vi "Configure Return Delay.vi"(8 "error in (no error)":errorcluster, 9 "Return Delay (500 microseconds)":sgl=500.0, 10 "Motor ID (0)":u8, 11 "Dynamixel Motor VISA in":refnum<class "Dynamixel Motor VISA.lvclass">) -> (0 "error out":errorcluster, 3 "Dynamixel Motor VISA out":refnum<class "Dynamixel Motor VISA.lvclass">)   [LabVIEW 2016, in "Dynamixel Motor VISA.lvclass"]
doc: "Sets the return delay time for the motor."
uses:
  <instrlib>/Dynamixel Motor/HAIOL/VISA/Dynamixel Motor VISA.lvclass
  <instrlib>/Dynamixel Motor/HAIOL/VISA/Dynamixel Motor VISA.lvclass/Dynamixel Motor VISA.ctl
  <instrlib>/Dynamixel Motor/Dynamixel Motor.lvlib
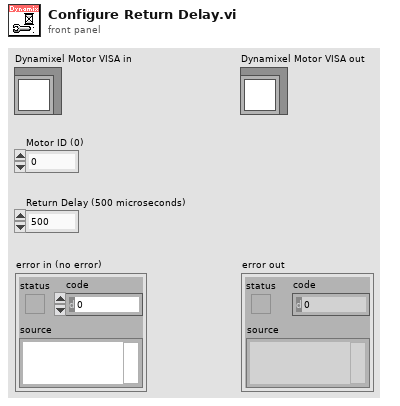
[diagram p1: front panel]
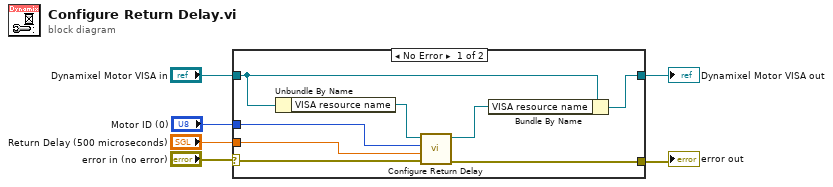
[diagram p0: block diagram]
diagram:
  n1 = case shown="No Error" "error in (no error)" {
    selector: "error in (no error)" -> [w11 w15]
    tunnel: "Dynamixel Motor VISA in" -> [w8 w16]
    tunnel: "Motor ID (0)" -> [w13 _]
    tunnel: "Return Delay (500 microseconds)" -> [w12 _]
    tunnel: [w10 w15] -> w2
    tunnel: [w7 w16] -> w1
    frame No Error {
      n2 = Unbundle By Name(w8) -> ("VISA resource name"=w14:refnum<visa-resource-name>)
      n3 = call <instrlib>:"Configure Return Delay.vi"("error in (no error)"=w11, "Return Delay (500 microseconds)"=w12, "Motor ID (0)"=w13, "VISA resource name"=w14) -> ("error out"=w10:errorcluster, "VISA resource name out"=w9:refnum<visa-resource-name>)  [unwired: 6 in]
      n4 = Bundle By Name(cluster=w8, "VISA resource name"=w9) -> (w7:refnum<class "Dynamixel Motor VISA.lvclass">)
    }
    frame Error {
    }
  }
  "error out" <- w2
  "Dynamixel Motor VISA out" <- w1
